vi "TestStopOutWaveBank.vi"(8 "error in (no error)":errorcluster) -> (0 "error out":errorcluster)   [LabVIEW 2020]
uses:
  <vilib>/addons/_JKI Toolkits/Caraya/classes/Test/Test.lvclass
  <vilib>/addons/_JKI Toolkits/Caraya/classes/Assert/Assert.lvclass
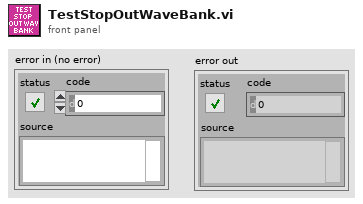
[diagram p1: front panel]
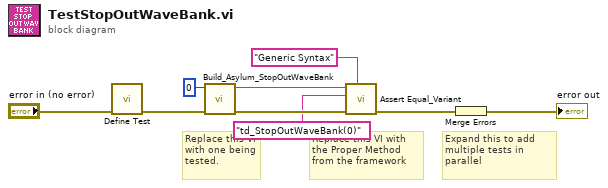
[diagram p0: block diagram]
diagram:
  # "Expand this to add multiple tests in parallel"
  # "Replace this VI with one being tested."
  # "Replace this VI with the Proper Method from the framework"
  n1 = call <vilib>:"Define Test.vi"("error in (no error)"="error in (no error)") -> ("error out"=w5:errorcluster)  [unwired: 10 in]
  n2 = call "Build_Asylum_StopOutWaveBank.vi"("error in (no error)"=w5, "whichBank"=0) -> ("error out"=w3:errorcluster, "Command"=w4:string)  [unwired: 8 in]
  n3 = call <vilib>:"Assert Equal_Variant.vi"("Label"="Generic Syntax", "error in (no error)"=w3, "Y"="td_StopOutWaveBank(0)", "X"=w4) -> ("error out"=w7:errorcluster)  [unwired: 7 in]
  n4 = Merge Errors(w7) -> (→"error out":errorcluster)
